vi "Open.vi"(8 "error in":errorcluster, 11 "Standard Engine in":refnum<class "Standard Engine Runtime.lvclass">) -> (0 "error out":errorcluster, 3 "Standard Engine out":refnum<class "Standard Engine Runtime.lvclass">)   [LabVIEW 2013, in "Standard Engine Runtime.lvclass"]
uses:
  Standard Engine Runtime.lvclass
  Commands.ctl
  Engine Config Data.ctl
  Configuration/Standard Engine Configuration.lvclass
  <vilib>/NI/Tag Bus Module Framework/runtime/TBM module execution interface.lvclass
  <vilib>/NI/Tag Bus Module Framework/module configuration/TBM module configuration.lvclass
  <vilib>/NI/Module Execution Interface/Engine Runtime/Execution States.ctl
  Engine Process Init Data.ctl
  Standard Engine Runtime.lvclass/Standard Engine Runtime.ctl
  <vilib>/NI/Module Execution Interface/Engine Runtime/Engine Runtime Interface.lvclass
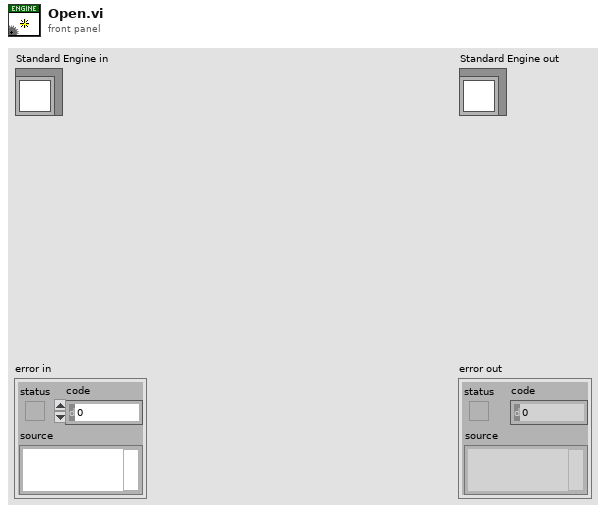
[diagram p1: front panel]
types:
  T1 = typedef "Engine Runtime Interface.lvclass/Execution States.ctl" = enum16{"Initializing", "Paused (Initialized)", "Running", "Set Safe Outputs", "Uninitializing", "Stopped (Uninitialized)", "Error (Uninitialized)", "Safe State (Uninitialized)", "Closed"}
  T2 = typedef "Standard Engine Runtime.lvclass/Engine Process Init Data.ctl" = cluster{"Messages FIFO":refnum<k33>, "Engine Config. Ref":refnum<data-value>, "Status Notifier":refnum<notifier>, "Error Queue":refnum<queue>}
  T3 = typedef "Standard Engine Runtime.lvclass/Engine Config Data.ctl" = cluster{"Engine Configuration":refnum<class "Standard Engine Configuration.lvclass">, "Modules":refnum<class "TBM module execution interface.lvclass">[], "Module Configurations":refnum<class "TBM module configuration.lvclass">[]}
  T4 = typedef "Standard Engine Runtime.lvclass/Commands.ctl" = enum16{"Initialize", "Start", "Pause", "Safe State", "Normal", "Stop", "Shutdown"}
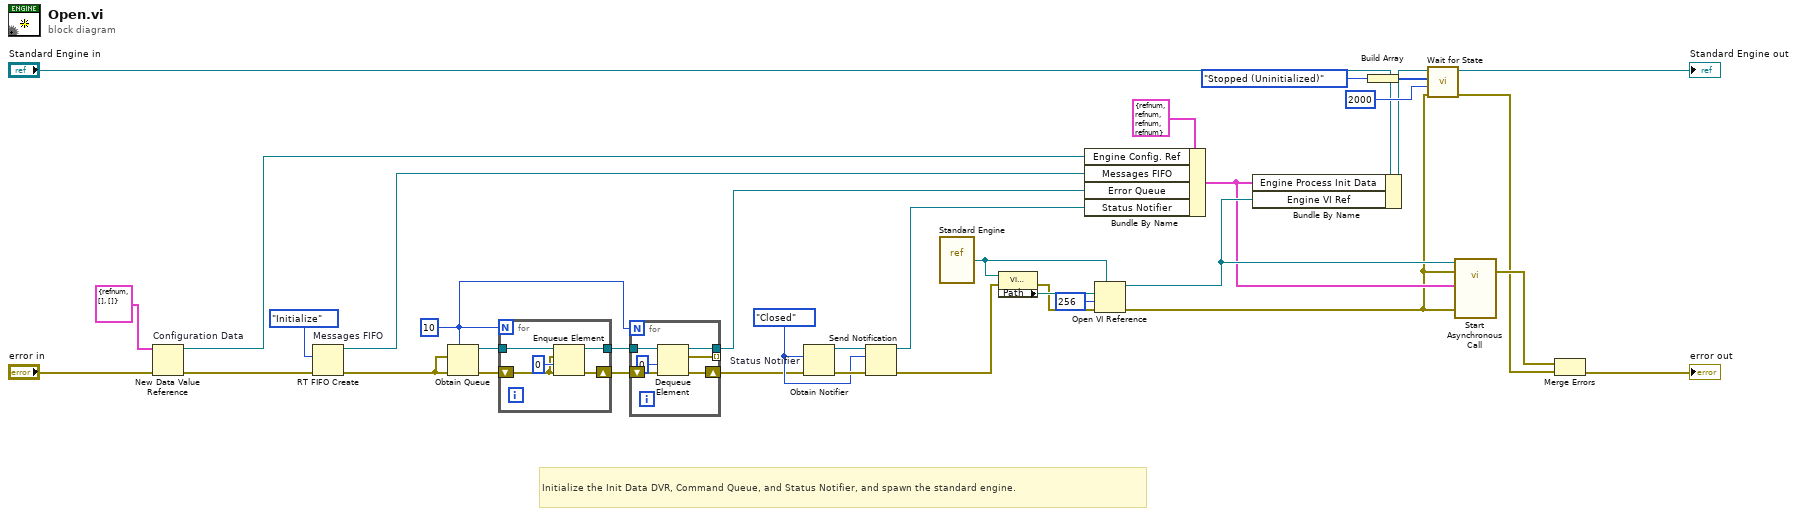
[diagram p0: block diagram]
diagram:
  w10 = 10 ("max queue size (-1, unlimited)")
  w26 = Execution_States."Closed" ("States")
  # "Initialize the Init Data DVR, Command Queue, and Status Notifier, and spawn the standard engine."
  n1 = New Data Value Reference "Configuration Data"(data value=T3 {"Engine Configuration"=refnum, "Modules"=[], "Module Configurations"=[]} ("Engine Configuration Data"), error in="error in") -> (data value reference=w21:refnum<data-value>, error out=w30:errorcluster)
  n2 = RT FIFO Create "Messages FIFO"(1:Commands."Initialize" ("Commands"), 3:w30) -> (8:w20:refnum<k33>, 11:w5:errorcluster)  [unwired: 6 in, 1 out]
  n3 = Obtain Queue(max queue size (-1, unlimited)=w10, element data type=w5, error in (no error)=w5) -> (queue out=w12:refnum<queue>, error out=w11:errorcluster)  [unwired: 2 in, 1 out]
  n4 = for {
    N: w10 -> [_]
    tunnel: w12 -> [w41]
    shift-right: [w40] -> w8
    shift-left: w11 -> [w37]
    tunnel: [w38] -> w9
    n5 = Enqueue Element(queue=w41, element=w37, timeout in ms (-1)=0, error in (no error)=w37) -> (queue out=w38:refnum<queue>, error out=w40:errorcluster)  [unwired: 1 out]
  }
  n6 = for {
    N: w10 -> [_]
    tunnel: w9 -> [w47]
    shift-right: [w45] -> w6
    shift-left: w8 -> [w46]
    tunnel: [w44] -> w7
    tunnel: [w42] -> _ mode=indexing
    n7 = Dequeue Element(queue=w47, timeout in ms (-1)=0, error in (no error)=w46) -> (queue out=w44:refnum<queue>, element=w42:errorcluster, error out=w45:errorcluster)  [unwired: 1 out]
  }
  n8 = Obtain Notifier "Status Notifier"(notification data type=w26, error in (no error)=w6) -> (notifier out=w27:refnum<notifier>, error out=w28:errorcluster)  [unwired: 2 in, 1 out]
  n9 = Send Notification(notification=w26, notifier=w27, error in (no error)=w28) -> (notifier out=w18:refnum<notifier>, error out=w25:errorcluster)
  n10 = vi-ref "Standard Engine.vi"() -> (w29:refnum<vi>)
  n11 = property class="VI (strict)"(reference=w29, error in=w25) -> (error out=w34:errorcluster, "Path"=w35:path)  [unwired: 1 out]
  n12 = Bundle By Name(cluster=T2 {"Messages FIFO"=refnum, "Engine Config. Ref"=refnum, "Status Notifier"=refnum, "Error Queue"=refnum} ("Engine Process Init Data"), "Engine Config. Ref"=w21, "Messages FIFO"=w20, "Error Queue"=w7, "Status Notifier"=w18) -> (w19:T2)
  n13 = Open VI Reference(type specifier VI Refnum (for type only)=w29, vi path=w35, options=256, error in (no error)=w34) -> (vi reference=w23:refnum<vi>, error out=w17:errorcluster)  [unwired: 2 in]
  n14 = Bundle By Name(cluster="Standard Engine in", "Engine Process Init Data"=w19, "Engine VI Ref"=w23) -> (w2:refnum<class "Standard Engine Runtime.lvclass">)
  n15 = Build Array(Execution_States."Stopped (Uninitialized)" ("notification")) -> (w14:T1[])
  n16 = call "Wait for State.vi"("error in"=w17, "timeout in ms"=2000, "expected states"=w14, "Standard Engine in"=w2) -> ("error out"=w3:errorcluster, "Standard Engine out"=→"Standard Engine out":refnum<class "Standard Engine Runtime.lvclass">)  [unwired: 6 in]
  n17 = call-by-ref "Start Asynchronous Call"(reference=w23, error in=w17, 8:"error in (no error)"=w17, "Engine Process Init Data"=w19) -> (error out=w24:errorcluster)  [unwired: 9 in, 2 out]
  n18 = Merge Errors(w24, w3) -> (→"error out":errorcluster)
